vi "Write stack report.vi"(8 "error in (no error)":errorcluster, 11 "Autofocus in":refnum<class "Autofocus.lvclass">) -> (0 "error out":errorcluster, 3 "Autofocus out":refnum<class "Autofocus.lvclass">)   [LabVIEW 2012, in "Autofocus.lvclass"]
uses:
  Autofocus.lvclass
  Autofocus.lvclass/Autofocus.ctl
  <vilib>/Utility/file.llb/Write To Spreadsheet File (string).vi
  <vilib>/Utility/file.llb/Write To Spreadsheet File (DBL).vi
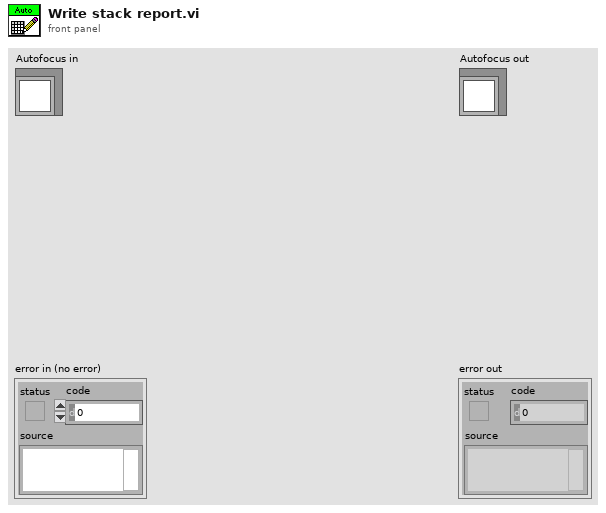
[diagram p1: front panel]
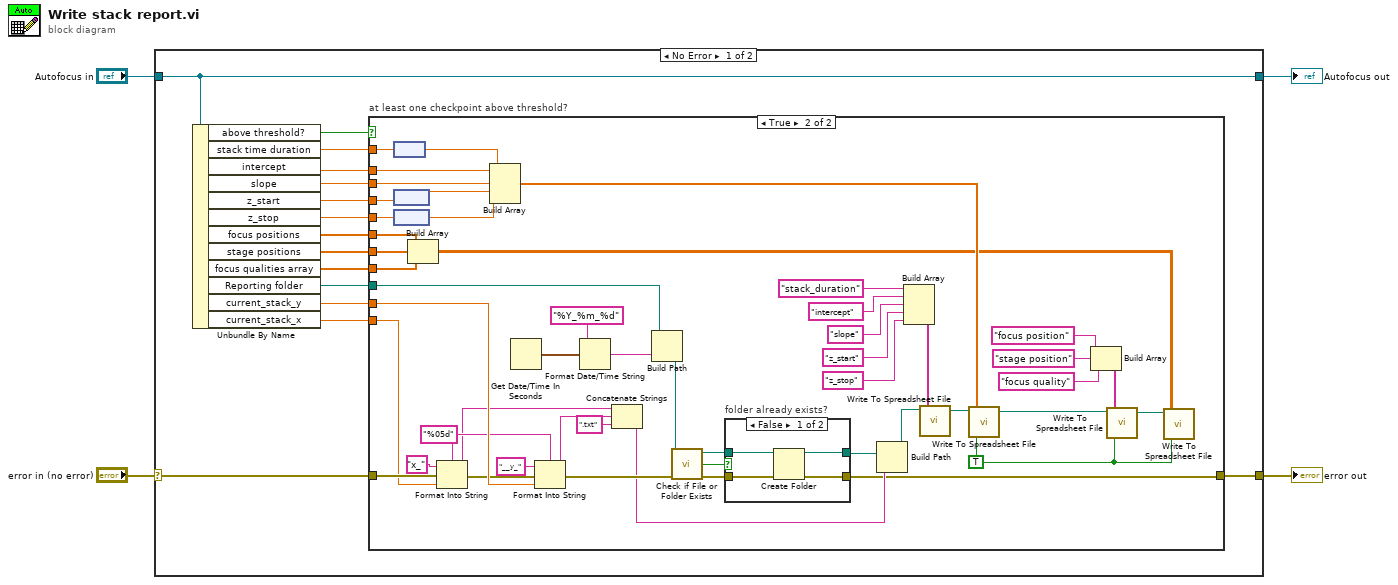
[diagram p0: block diagram]
diagram:
  n1 = case shown="No Error" "error in (no error)" {
    selector: "error in (no error)" -> [w18 w78]
    tunnel: [w17 w78] -> w3
    tunnel: [w19 w77] -> w1
    tunnel: "Autofocus in" -> [w19 w77]
    frame No Error {
      n2 = Unbundle By Name(w19) -> ("above threshold?"=w6:bool, "stack time duration"=w5:dbl[unit], "intercept"=w10:dbl, "slope"=w9:dbl, "z_start"=w8:dbl[unit], "z_stop"=w7:dbl[unit], "focus positions"=w12:dbl[], "stage positions"=w13:dbl[], "focus qualities array"=w14:dbl[], "Reporting folder"=w11:path, "current_stack_y"=w15:dbl[unit], "current_stack_x"=w16:dbl[unit])
      n3 = case "at least one checkpoint above threshold?" shown="True" w6 {
        tunnel: w18 -> [w20 w70]
        tunnel: [w20 w45] -> w17
        tunnel: w16 -> [_ w69]
        tunnel: w15 -> [_ w68]
        tunnel: w14 -> [_ w63]
        tunnel: w13 -> [_ w62]
        tunnel: w12 -> [_ w61]
        tunnel: w11 -> [_ w55]
        tunnel: w10 -> [_ w34]
        tunnel: w9 -> [_ w33]
        tunnel: w8 -> [_ w32]
        tunnel: w7 -> [_ w31]
        tunnel: w5 -> [_ w23]
        frame False {
        }
        frame True {
          w24 = TRUE ("append to file? (new file:F)")
          w64 = "%05d" ("format string")
          n4 = node(w23) -> (w22:dbl)
          n5 = node(w32) -> (w30:dbl)
          n6 = node(w31) -> (w29:dbl)
          n7 = Build Array(w61, w62, w63) -> (w25:dbl[][])
          n8 = Format Into String(format string=w64, initial string="x_", error in=w70, w69) -> (resulting string=w60:string, error out=w67:errorcluster)
          n9 = Build Array(w22, w34, w33, w30, w29) -> (w28:dbl[])
          n10 = Get Date/Time In Seconds() -> (seconds since 1Jan1904=w57:timestamp)
          n11 = Format Into String(format string=w64, initial string="__y_", error in=w67, w68) -> (resulting string=w59:string, error out=w53:errorcluster)
          n12 = Format Date/Time String(time format string (%c)="%Y_%m_%d", seconds (now)=w57) -> (date/time string=w54:string)  [unwired: 1 in]
          n13 = Concatenate Strings(w60, w59, ".txt" ("string")) -> (w47:string)
          n14 = Build Path(base path=w55, name or relative path=w54) -> (appended path=w52:path)
          n15 = call <vilib>:"Check if File or Folder Exists.vi"("error in (no error)"=w53, "path"=w52) -> ("error out"=w50:errorcluster, "file or folder exists?"=w51:bool, "dup path"=w49:path)  [unwired: 7 in]
          n16 = case "folder already exists?" shown="False" w51 {
            tunnel: [w72 w76] -> w45
            tunnel: w50 -> [w74 w76]
            tunnel: w49 -> [w73 w75]
            tunnel: [w71 w75] -> w48
            frame False {
              n17 = Create Folder(path (use dialog)=w73, error in=w74) -> (created path=w71:path, error out=w72:errorcluster)  [unwired: 1 in, 1 out]
            }
            frame True {
            }
          }
          n18 = Build Path(base path=w48, name or relative path=w47) -> (appended path=w46:path)
          n19 = Build Array("stack_duration" ("string"), "intercept" ("string"), "slope" ("string"), "z_start" ("string"), "z_stop" ("string")) -> (w37:string[])
          n20 = call-poly <vilib>:"Write To Spreadsheet File.vi"("1D data"=w37, "file path (dialog if empty)"=w46) -> ("new file path (Not A Path if cancelled)"=w35:path)  [unwired: 6 in]
          n21 = call-poly <vilib>:"Write To Spreadsheet File.vi"("append to file? (new file:F)"=w24, "1D data"=w28, "file path (dialog if empty)"=w35) -> ("new file path (Not A Path if cancelled)"=w27:path)  [unwired: 5 in]
          n22 = Build Array("focus position" ("string"), "stage position" ("string"), "focus quality" ("string")) -> (w26:string[])
          n23 = call-poly <vilib>:"Write To Spreadsheet File.vi"("append to file? (new file:F)"=w24, "1D data"=w26, "file path (dialog if empty)"=w27) -> ("new file path (Not A Path if cancelled)"=w36:path)  [unwired: 5 in]
          n24 = call-poly <vilib>:"Write To Spreadsheet File.vi"("append to file? (new file:F)"=w24, "2D data"=w25, "file path (dialog if empty)"=w36) -> ()  [unwired: 5 in, 1 out]
        }
      }
    }
    frame Error {
    }
  }
  "error out" <- w3
  "Autofocus out" <- w1
